vi "Compute RT Index from Label and SDI.vi"(10 "SDI":u8 format="%0d", 11 "label":u8) -> (3 "RT label index":i32 format="%0d")   [LabVIEW 2020, in "AIM ARINC 429 Engine.lvlib" / "Custom Device.lvlib"]
uses:
  Custom Device.lvlib
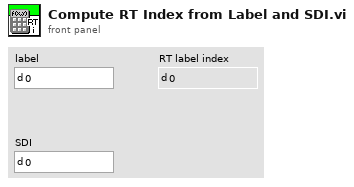
[diagram p1: front panel]
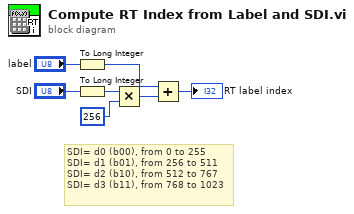
[diagram p0: block diagram]
diagram:
  # "SDI= d0 (b00), from 0 to 255\nSDI= d1 (b01), from 256 to 511\nSDI= d2 (b10), from 512 to 767\nSDI= d3 (b11), from 768 to 1023"
  n1 = To Long Integer(number="label") -> (32bit integer=w7:i32)
  n2 = To Long Integer(number="SDI") -> (32bit integer=w4:i32)
  n3 = Multiply(x=w4, y=256) -> (x*y=w5:i32)
  n4 = Add(x=w7, y=w5) -> (x+y=→"RT label index":i32)
